vi "Quick Usb Get Last Error.vi"(8 "error in (no error)":errorcluster, 11 "error":u32) -> (0 "error out":u32, 2 "function return":i32, 3 "error out 2":errorcluster)   [LabVIEW 2011, in "QuickUSB.lvlib"]
doc: "QUSBLIB QRETURN QuickUsbGetLastError(\n PQULONG error\n);"
uses:
  QuickUSB.lvlib
  QuickUSB.dll
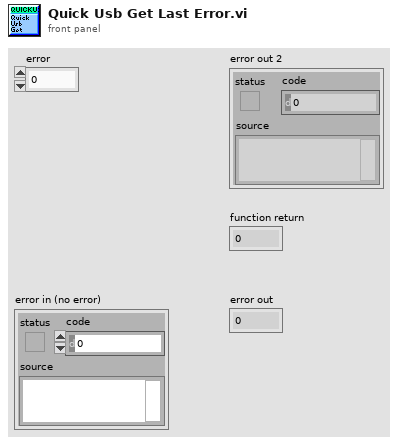
[diagram p1: front panel]
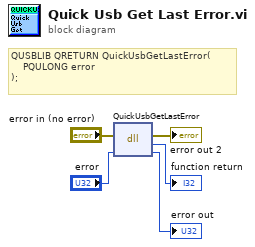
[diagram p0: block diagram]
diagram:
  # "QUSBLIB QRETURN QuickUsbGetLastError(\n    PQULONG error\n);"
  n1 = dll-call lib="C:/QuickUSB/QuickUSB.*" fn="QuickUsbGetLastError"(error in="error in (no error)", "error"="error") -> (error out=→"error out 2":errorcluster, →"function return":i32, "error"=→"error out":u32)  [unwired: 2 in, 1 out]
